vi "路径.vi"(11 "输入路径":path) -> (3 "输出路径":path)   [LabVIEW 2015]
panel:
  out "名称":string
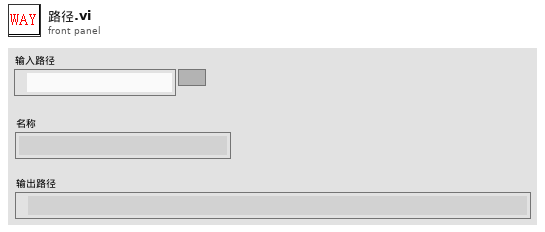
[diagram p1: front panel]
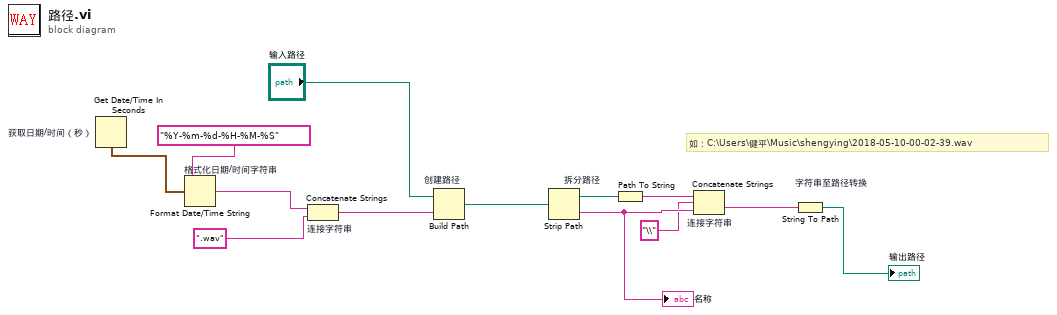
[diagram p0: block diagram]
diagram:
  # "如：C:\\Users\\健平\\Music\\shengying\\2018-05-10-00-02-39.wav"
  n1 = Get Date/Time In Seconds "获取日期/时间（秒）"() -> (seconds since 1Jan1904=w10:timestamp)
  n2 = Format Date/Time String "格式化日期/时间字符串"(time format string (%c)="%Y-%m-%d-%H-%M-%S", seconds (now)=w10) -> (date/time string=w12:string)  [unwired: 1 in]
  n3 = Concatenate Strings "连接字符串"(w12, ".wav" ("元素")) -> (w8:string)
  n4 = Build Path "创建路径"(base path="输入路径", name or relative path=w8) -> (appended path=w13:path)
  n5 = Strip Path "拆分路径"(path=w13) -> (stripped path=w6:path, name=w5:string)
  "名称" <- w5
  n6 = Path To String(path=w6) -> (string=w3:string)
  n7 = Concatenate Strings "连接字符串"(w3, "\\" ("字符串"), w5) -> (w7:string)
  n8 = String To Path "字符串至路径转换"(string=w7) -> (path=→"输出路径":path)
